vi "Create run.vi"(8 "error in (no error)":errorcluster, 9 "all rows":string[][](array[string]), 10 "Which group":i32=1, 11 "number of samples between standards":i32=4) -> (0 "error out":errorcluster, 1 "Group run list":string[][](array[string]))   [LabVIEW 2016]
doc: "This vi takes the 2d array from a wheel file and creates a group run list"
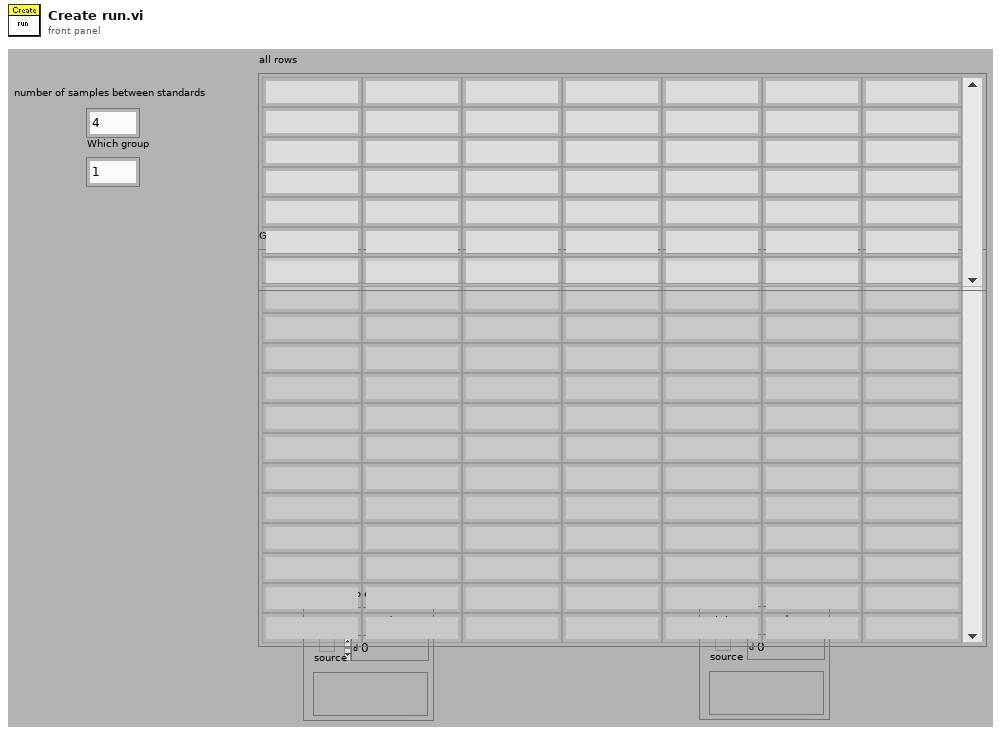
[diagram p1: front panel]
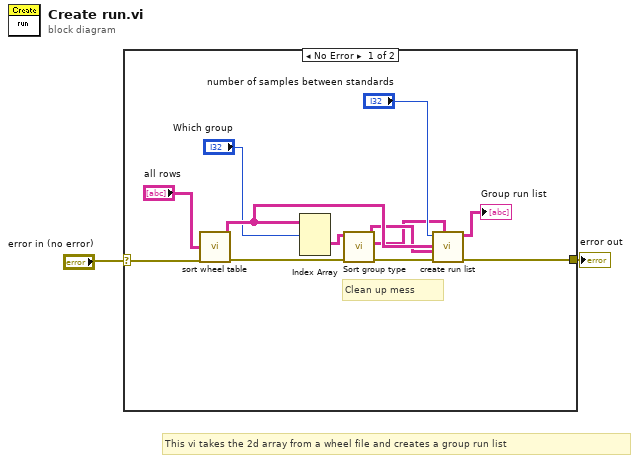
[diagram p0: block diagram]
diagram:
  # "This vi takes the 2d array from a wheel file and creates a group run list"
  n1 = case shown="No Error" "error in (no error)" {
    selector: "error in (no error)" -> [w4 w15]
    tunnel: [w3 w15] -> w1
    frame No Error {
      # "Clean up mess"
      n2 = call "sort wheel table.vi"("Wheel table"="all rows", "error in (no error)"=w4) -> ("Paged groups"=w11:string[][][], "error out"=w8:errorcluster)  [unwired: 12 out]
      n3 = Index Array(array=w11, index (dim 0)="Which group") -> (element=w7:string[][])  [unwired: 2 in]
      n4 = call "Sort group type.vi"("error in (no error)"=w8, "Paged groups"=w7) -> ("error out"=w13:errorcluster, "Group Stanards"=w9:string[][], "Group Unknowns"=w10:string[][])  [unwired: 7 out]
      n5 = call "create run list.vi"("Group Stanards"=w9, "error in (no error)"=w13, "Group Unknowns"=w10, "Paged groups"=w11, "number of samples between standards"="number of samples between standards") -> ("error out"=w3:errorcluster, "Group run list"=→"Group run list":string[][])  [unwired: 1 in, 4 out]
    }
    frame Error {
    }
  }
  "error out" <- w1
